vi "IsMaster.vi"(8 "error in (no error)":errorcluster, 11 "Network Slave in":refnum<class "Network Slave.lvclass">) -> (0 "error out":errorcluster, 2 "isMaster":bool, 3 "Network Slave out":refnum<class "Network Slave.lvclass">)   [LabVIEW 2020, in "SubVIs.lvlib" / "Network Slave.lvclass"]
uses:
  <vilib>/Modbus/subvis/Protocol/Interfaces/Network Slave/Network Slave.lvclass
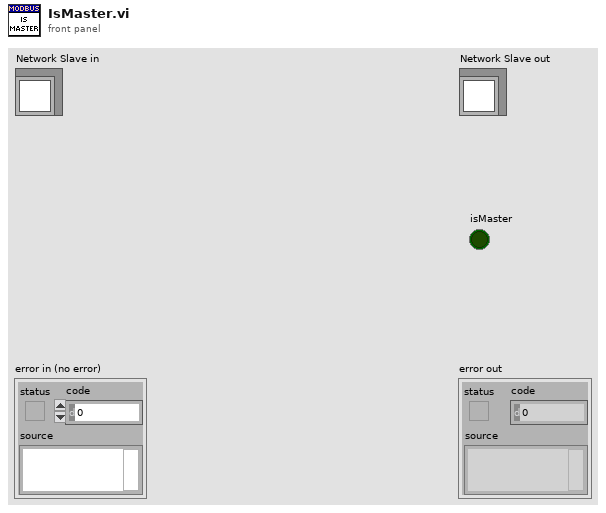
[diagram p1: front panel]
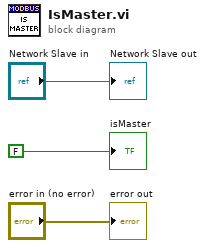
[diagram p0: block diagram]
diagram:
  "error out" <- "error in (no error)"
  "Network Slave out" <- "Network Slave in"
  "isMaster" <- FALSE ("isMaster")
